vi "VI Server Setup.vi"(9 "This VI":refnum<vi>, 10 "This Application":refnum<vi>, 11 "TEMPLATE jettl in":refnum<class "TEMPLATE jettl.lvclass">) -> (3 "TEMPLATE jettl out":refnum<class "TEMPLATE jettl.lvclass">)   [LabVIEW 2021, in "_Template.lvlib" / "Templates.lvlib" / "TEMPLATE jettl.lvlib" / "TEMPLATE jettl.lvclass"]
uses:
  TEMPLATE jettl.lvclass
  TEMPLATE jettl.lvclass/TEMPLATE jettl.ctl
  jettl/jettl/jettl/jettl.lvclass
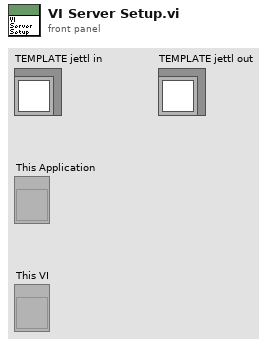
[diagram p1: front panel]
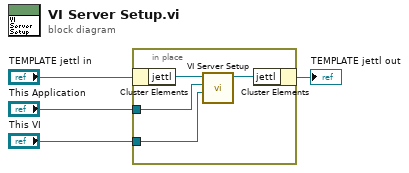
[diagram p0: block diagram]
diagram:
  n1 = in-place {
    in-place-border: "This Application" -> [w6]
    in-place-border: "This VI" -> [w5]
    n2 = in-place-cluster #1("TEMPLATE jettl in") -> ("jettl"=w8:refnum<class "jettl.lvclass">)
    n3 = call-dynamic "VI Server Setup.vi"("This VI"=w5, "This Application"=w6, "jettl in"=w8) -> ("jettl out"=w7:refnum<class "jettl.lvclass">)  [unwired: 8 in]
    n4 = in-place-cluster #1("jettl"=w7) -> (→"TEMPLATE jettl out":refnum<class "TEMPLATE jettl.lvclass">)
  }
